vi "send_trajectory.vi"(8 "error in (no error)":errorcluster, 10 "trajectory":refnum<class "GenericTrajectory.lvclass">, 11 "GenericScanHead in":refnum<class "GenericScanHead.lvclass">) -> (0 "error out":errorcluster, 3 "GenericScanHead out":refnum<class "GenericScanHead.lvclass">)   [LabVIEW 2010, in "GenericScanHead.lvclass"]
uses:
  GenericScanHead.lvclass
  Trajectory/GenericTrajectory/GenericTrajectory/GenericTrajectory.lvclass
  trigger_enum.ctl
  class_data.vi
  common/classes/ErrorController/ErrorController/class_data.vi
  common/classes/ErrorController/ErrorController/ErrorController.lvclass
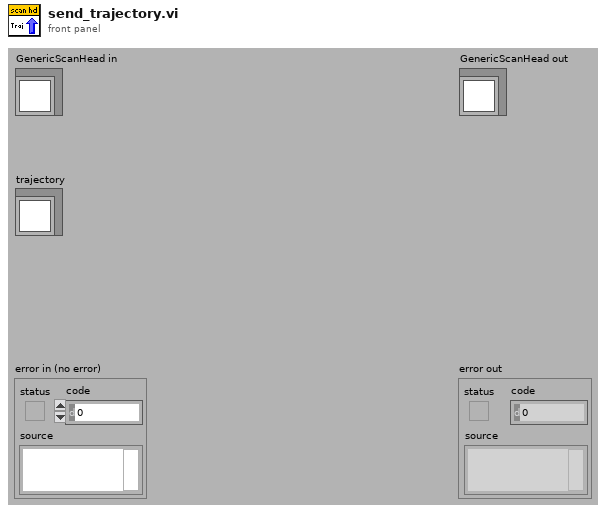
[diagram p1: front panel]
types:
  T1 = typedef "GenericScanHead.lvclass/trigger_enum.ctl" = enum16{"NULL", "fetch trajectory", "generate trajectory", "change run mode", "update modifiers"}
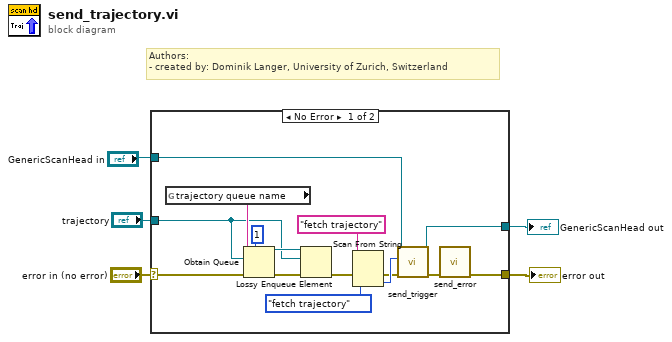
[diagram p0: block diagram]
diagram:
  # "Authors: \n- created by: Dominik Langer, University of Zurich, Switzerland"
  n1 = case shown="No Error" "error in (no error)" {
    selector: "error in (no error)" -> [w19 w22]
    tunnel: [w12 w22] -> w4
    tunnel: [w16 w21] -> w2
    tunnel: "GenericScanHead in" -> [w17 w21]
    tunnel: "trajectory" -> [w14 _]
    frame No Error {
      n2 = global read "class_data.vi" "trajectory queue name"() -> (w18:string)
      n3 = Obtain Queue(max queue size (-1, unlimited)=1, name (unnamed)=w18, element data type=w14, error in (no error)=w19) -> (queue out=w20:refnum<queue>, error out=w15:errorcluster)  [unwired: 1 in, 1 out]
      n4 = Lossy Enqueue Element(queue=w20, element=w14, error in (no error)=w15) -> (error out=w9:errorcluster)  [unwired: 3 out]
      n5 = Scan From String(input string="fetch trajectory", error in=w9, default 1=trigger_enum."fetch trajectory" ("trigger")) -> (error out=w8:errorcluster, output 1=w10:T1)  [unwired: 2 in, 2 out]
      n6 = call-dynamic "send_trigger.vi"("error in (no error)"=w8, "trigger"=w10, "GenericScanHead in"=w17) -> ("error out"=w13:errorcluster, "GenericScanHead out"=w16:refnum<class "GenericScanHead.lvclass">)  [unwired: 7 out]
      n7 = call "send_error.vi"("error in (no error)"=w13) -> ("error out"=w12:errorcluster)  [unwired: 10 in]
    }
    frame Error {
    }
  }
  "error out" <- w4
  "GenericScanHead out" <- w2
